vi "Load_Comparitor_Cluster.vi"() -> ()   [LabVIEW 2011]
uses:
  ADAM_Comparitor.ctl
  Anemometry/Anemometry Sub Vis/Globals/Constants_global.vi
  ADAM_Global.vi
panel:
  out "Channel Values Out":string[][](array[string])
  out "Ch names Out":string[](array[string])
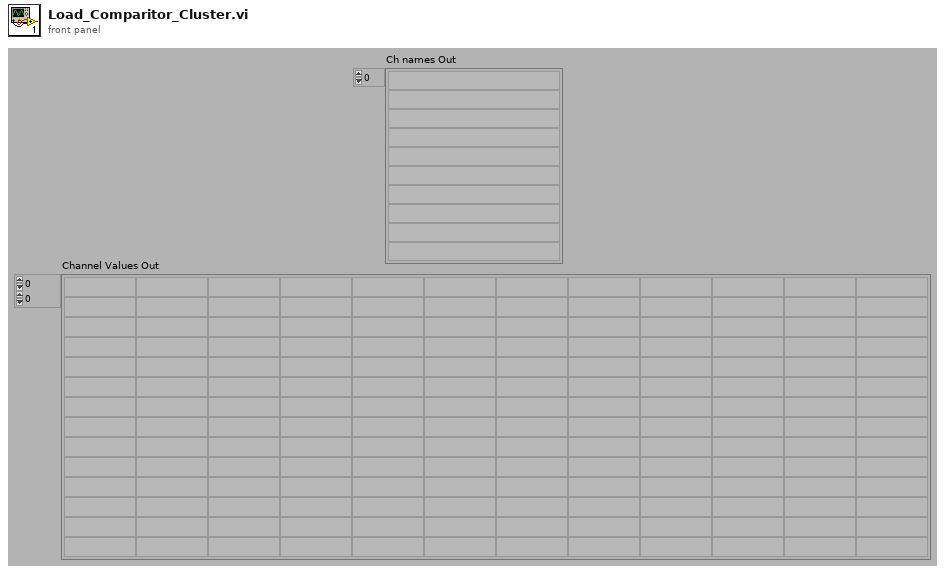
[diagram p1: front panel]
types:
  T1 = typedef "ADAM_Comparitor.ctl" = cluster{"Ch to Monitor":string, "Channels to Kill":string, "Warn if Above":dbl, "Warn if Below":dbl, "Kill if Above":dbl, "Kill if Below":dbl, "Hysteresis Margin":dbl, "Averaging TIme (s)":dbl, "Warn Status":bool, "Kill Status":bool, "Extra Email addresses":string}
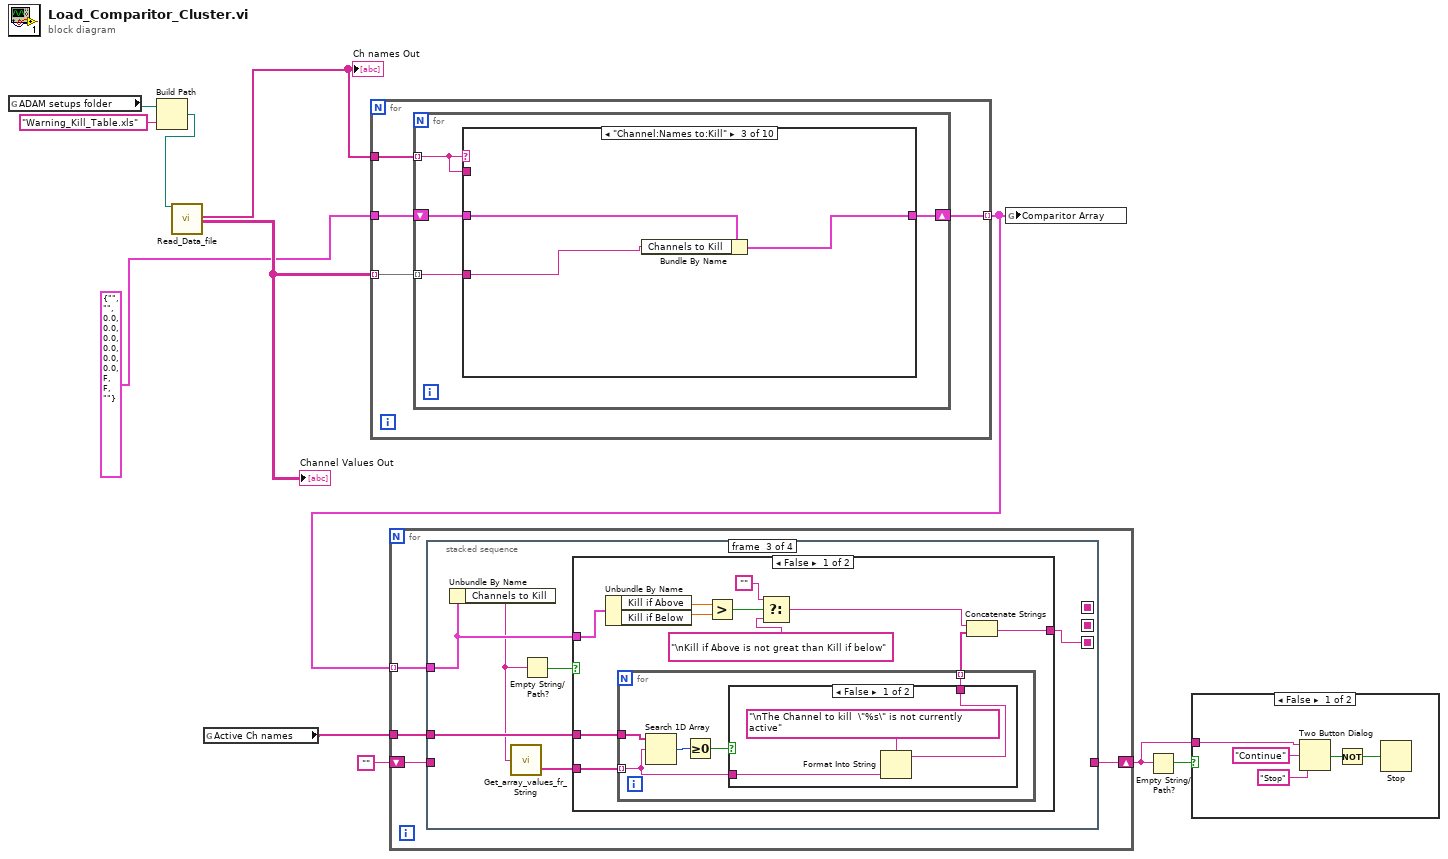
[diagram p0: block diagram]
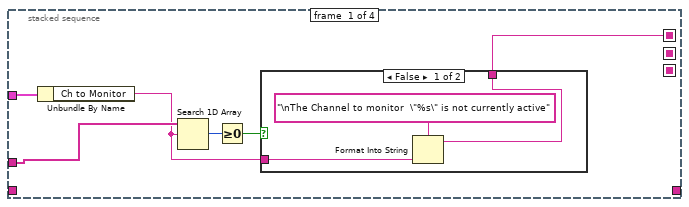
[diagram p3: hidden frame]
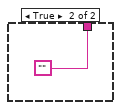
[diagram p4: hidden frame]
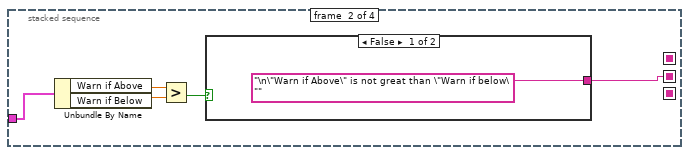
[diagram p5: hidden frame]
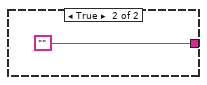
[diagram p6: hidden frame]
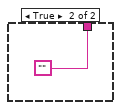
[diagram p7: hidden frame]
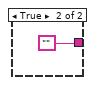
[diagram p8: hidden frame]
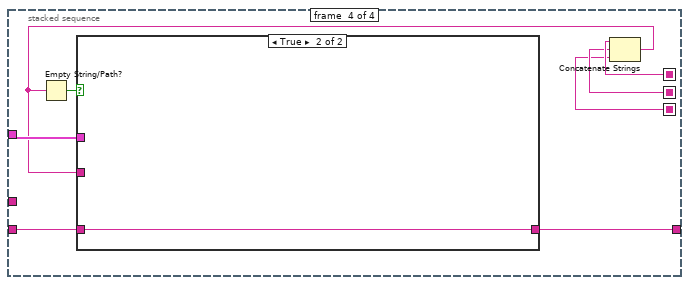
[diagram p9: hidden frame]
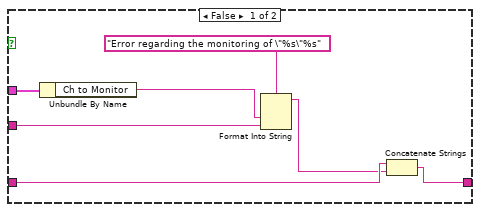
[diagram p10: hidden frame]
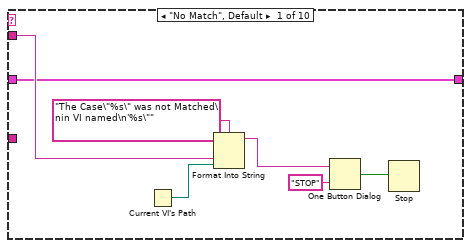
[diagram p11: hidden frame]
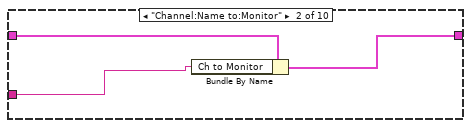
[diagram p12: hidden frame]
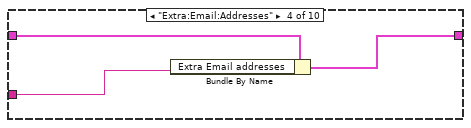
[diagram p13: hidden frame]
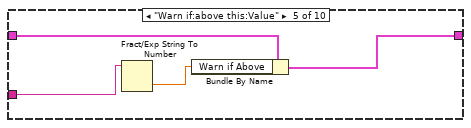
[diagram p14: hidden frame]
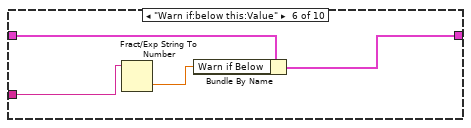
[diagram p15: hidden frame]
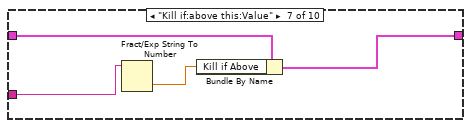
[diagram p16: hidden frame]
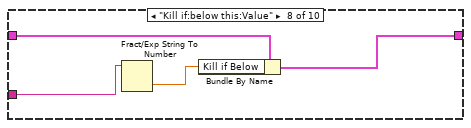
[diagram p17: hidden frame]
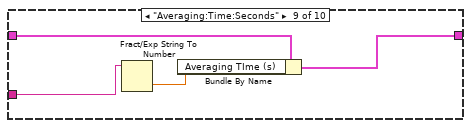
[diagram p18: hidden frame]
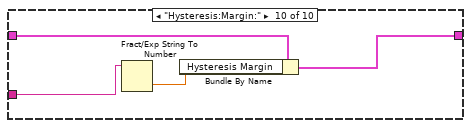
[diagram p19: hidden frame]
diagram:
  n1 = global read "Constants_global.vi" "ADAM setups folder"() -> (w4:path)
  n2 = Build Path(base path=w4, name or relative path="Warning_Kill_Table.xls") -> (appended path=w2:path)
  n3 = call "Read_Data_file.vi"("Results file"=w2) -> ("Ch names Out"=w11:string[], "Channel Values Out"=w10:string[][])  [unwired: 9 in, 8 out]
  "Ch names Out" <- w11
  "Channel Values Out" <- w10
  n4 = global read "ADAM_Global.vi" "Active Ch names"() -> (w1:string[])
  n5 = for {
    tunnel: w11 -> [w15]
    tunnel: w10 -> [w14] mode=indexing
    tunnel: T1 {"Ch to Monitor"="", "Channels to Kill"="", "Warn if Above"=0.0, "Warn if Below"=0.0, "Kill if Above"=0.0, "Kill if Below"=0.0, "Hysteresis Margin"=0.0, "Averaging TIme (s)"=0.0, "Warn Status"=FALSE, "Kill Status"=FALSE, "Extra Email addresses"=""} ("Cluster") -> [w13]
    tunnel: [w12] -> w8 mode=indexing
    n6 = for {
      tunnel: w15 -> [w16] mode=indexing
      shift-right: [w18] -> w12
      shift-left: w13 -> [w17]
      tunnel: w14 -> [w19] mode=indexing
      n7 = case shown="\"Channel:Names to:Kill\"" w16 {
        tunnel: w19 -> [_ w29 w32 w35 w37 w41 w45 w49 w53 w57]
        tunnel: [w20 w28 w31 w34 w39 w43 w47 w51 w55 w59] -> w18
        tunnel: w17 -> [w20 w27 w30 w33 w38 w42 w46 w50 w54 w58]
        tunnel: w16 -> [w21 _ _ _ _ _ _ _ _ _]
        frame "No Match", Default {
          n8 = Current VI's Path() -> (path=w22:path)
          n9 = Format Into String(format string="The Case\"%s\" was not Matched\nin VI named\n'%s\"" ("Format String"), w21, w22) -> (resulting string=w25:string)  [unwired: 2 in, 1 out]
          n10 = One Button Dialog(message=w25, button name ("OK")="STOP") -> (true=w23:bool)
          n11 = Stop(stop? (T)=w23) -> ()
        }
        frame "Channel:Name to:Monitor" {
          n12 = Bundle By Name(cluster=w27, "Ch to Monitor"=w29) -> (w28:T1)
        }
        frame "Channel:Names to:Kill" {
          n13 = Bundle By Name(cluster=w30, "Channels to Kill"=w32) -> (w31:T1)
        }
        frame "Extra:Email:Addresses" {
          n14 = Bundle By Name(cluster=w33, "Extra Email addresses"=w35) -> (w34:T1)
        }
        frame "Warn if:above this:Value" {
          n15 = Fract/Exp String To Number(string=w37) -> (number=w36:dbl)  [unwired: 3 in, 1 out]
          n16 = Bundle By Name(cluster=w38, "Warn if Above"=w36) -> (w39:T1)
        }
        frame "Warn if:below this:Value" {
          n17 = Fract/Exp String To Number(string=w41) -> (number=w40:dbl)  [unwired: 3 in, 1 out]
          n18 = Bundle By Name(cluster=w42, "Warn if Below"=w40) -> (w43:T1)
        }
        frame "Kill if:above this:Value" {
          n19 = Fract/Exp String To Number(string=w45) -> (number=w44:dbl)  [unwired: 3 in, 1 out]
          n20 = Bundle By Name(cluster=w46, "Kill if Above"=w44) -> (w47:T1)
        }
        frame "Kill if:below this:Value" {
          n21 = Fract/Exp String To Number(string=w49) -> (number=w48:dbl)  [unwired: 3 in, 1 out]
          n22 = Bundle By Name(cluster=w50, "Kill if Below"=w48) -> (w51:T1)
        }
        frame "Averaging:Time:Seconds" {
          n23 = Fract/Exp String To Number(string=w53) -> (number=w52:dbl)  [unwired: 3 in, 1 out]
          n24 = Bundle By Name(cluster=w54, "Averaging TIme (s)"=w52) -> (w55:T1)
        }
        frame "Hysteresis:Margin:" {
          n25 = Fract/Exp String To Number(string=w57) -> (number=w56:dbl)  [unwired: 3 in, 1 out]
          n26 = Bundle By Name(cluster=w58, "Hysteresis Margin"=w56) -> (w59:T1)
        }
      }
    }
  }
  n27 = for {
    tunnel: w8 -> [w63] mode=indexing
    shift-right: [w60] -> w5
    shift-left: "" -> [w61]
    tunnel: w1 -> [w62]
    n28 = stacked-sequence {
      seq-local: [_ w78 _ _] -> [_ _ _ w114]
      seq-local: [_ _ w84 _] -> [_ _ _ w113]
      seq-local: [w64 _ _ _] -> [_ _ _ w115]
      tunnel: w63 -> [w68 w74 w85 w111]
      tunnel: w62 -> [w67 _ w83 _]
      tunnel: w61 -> [_ _ _ w109]
      tunnel: [_ _ _ w108] -> w60
      frame #0 {
        n29 = Unbundle By Name(w68) -> ("Ch to Monitor"=w65:string)
        n30 = Search 1D Array(1D array=w67, element=w65) -> (index of element=w66:i32)  [unwired: 1 in]
        n31 = Greater Or Equal To 0?(x=w66) -> (x >= 0?=w69:bool)
        n32 = case shown="False" w69 {
          tunnel: w65 -> [w72 _]
          tunnel: [w70 ""] -> w64
          frame False {
            n33 = Format Into String(format string="\nThe Channel to monitor  \"%s\" is not currently active", w72) -> (resulting string=w70:string)  [unwired: 2 in, 1 out]
          }
          frame True {
          }
        }
      }
      frame #1 {
        n34 = Unbundle By Name(w74) -> ("Warn if Above"=w77:dbl, "Warn if Below"=w76:dbl)
        n35 = Greater?(x=w77, y=w76) -> (0:w75:bool)
        n36 = case shown="False" w75 {
          tunnel: ["\n\"Warn if Above\" is not great than \"Warn if below\"" ""] -> w78
          frame False {
          }
          frame True {
          }
        }
      }
      frame #2 {
        n37 = Unbundle By Name(w85) -> ("Channels to Kill"=w82:string)
        n38 = call "Get_array_values_fr_String.vi"("String Value"=w82) -> ("String array"=w81:string[])  [unwired: 1 out]
        n39 = Empty String/Path?(string/path=w82) -> (empty?=w86:bool)
        n40 = case shown="False" w86 {
          tunnel: w85 -> [w97 _]
          tunnel: [w88 ""] -> w84
          tunnel: w83 -> [w94 _]
          tunnel: w81 -> [w87 _]
          frame False {
            n41 = Unbundle By Name(w97) -> ("Kill if Above"=w96:dbl, "Kill if Below"=w95:dbl)
            n42 = for {
              tunnel: w94 -> [w102]
              tunnel: [w99] -> w90 mode=indexing
              tunnel: w87 -> [w98] mode=indexing
              n43 = Search 1D Array(1D array=w102, element=w98) -> (index of element=w101:i32)  [unwired: 1 in]
              n44 = Greater Or Equal To 0?(x=w101) -> (x >= 0?=w100:bool)
              n45 = case shown="False" w100 {
                tunnel: w98 -> [w105 _]
                tunnel: [w103 ""] -> w99
                frame False {
                  n46 = Format Into String(format string="\nThe Channel to kill  \"%s\" is not currently active", w105) -> (resulting string=w103:string)  [unwired: 2 in, 1 out]
                }
                frame True {
                }
              }
            }
            n47 = Greater?(x=w96, y=w95) -> (0:w93:bool)
            n48 = Select(t="", s=w93, f="\nKill if Above is not great than Kill if below") -> (s? t:f=w89:string)
            n49 = Concatenate Strings(w89, w90) -> (w88:string)
          }
          frame True {
          }
        }
      }
      frame #3 {
        n50 = Concatenate Strings(w115, w114, w113) -> (w110:string)
        n51 = Empty String/Path?(string/path=w110) -> (empty?=w112:bool)
        n52 = case shown="True" w112 {
          tunnel: w111 -> [w122 _]
          tunnel: w110 -> [w119 _]
          tunnel: w109 -> [w118 w123]
          tunnel: [w116 w123] -> w108
          frame False {
            n53 = Unbundle By Name(w122) -> ("Ch to Monitor"=w121:string)
            n54 = Format Into String(format string="Error regarding the monitoring of \"%s\"%s", w121, w119) -> (resulting string=w117:string)  [unwired: 2 in, 1 out]
            n55 = Concatenate Strings(w118, w117) -> (w116:string)
          }
          frame True {
          }
        }
      }
    }
  }
  n56 = global write "ADAM_Global.vi" "Comparitor Array"(w8) -> ()
  n57 = Empty String/Path?(string/path=w5) -> (empty?=w6:bool)
  n58 = case shown="False" w6 {
    tunnel: w5 -> [w124 _]
    frame False {
      n59 = Two Button Dialog(message=w124, 1:"Stop" ("F button name (\"Cancel\")"), 2:"Continue" ("T button name (\"OK\")")) -> (T button?=w126:bool)
      n60 = Not(x=w126) -> (.not. x?=w125:bool)
      n61 = Stop(stop? (T)=w125) -> ()
    }
    frame True {
    }
  }
